vi "Post_Process_Measurement.vi"(1 "Raw data file":path) -> ()   [LabVIEW 2011]
uses:
  Controls/Setup.ctl
  Controls/Post_Process.ctl
  Controls/Save_Data.ctl
  Globals/Constants_global.vi
  Globals/Dynamic_call_global.ph.vi
panel:
  in  "User Specific":refnum<vi>
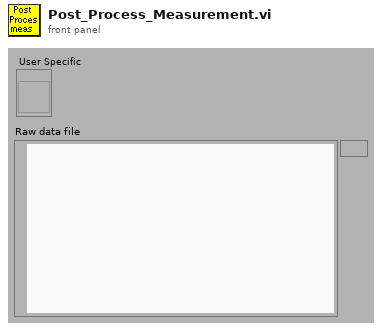
[diagram p1: front panel]
types:
  T1 = enum32{"Bad", "Idle", "Run top level", "Running"}
  T2 = typedef "Setup.ctl" = enum16{"Run Program", "Show Setup", "Save Current Setup", "Setup Front Panel"}
  T3 = typedef "Post_Process.ctl" = enum16{"Take New Data", "Post Process Raw Data File"}
  T4 = typedef "Save_Data.ctl" = enum16{"Save No Data", "Save Data"}
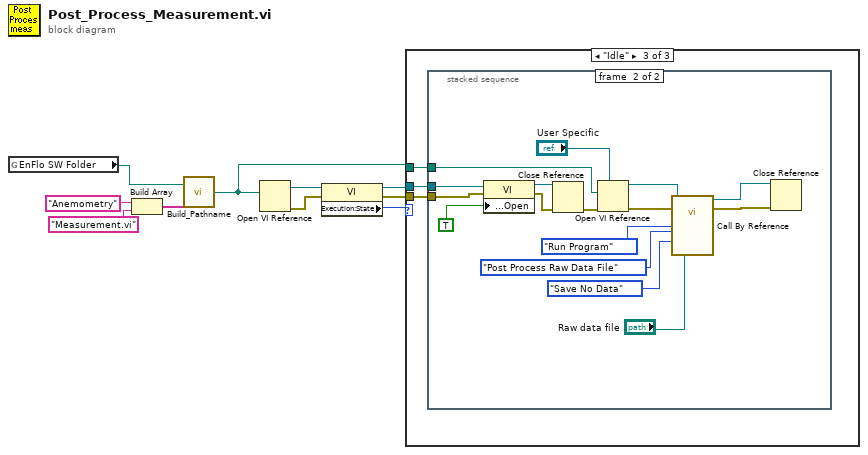
[diagram p0: block diagram]
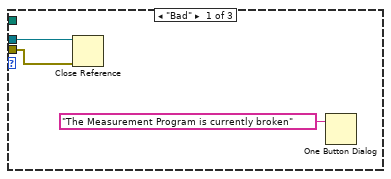
[diagram p2: hidden frame]
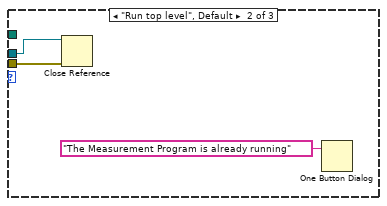
[diagram p3: hidden frame]
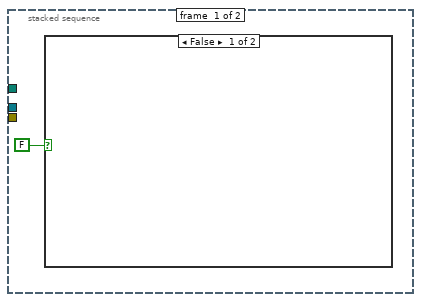
[diagram p4: hidden frame]
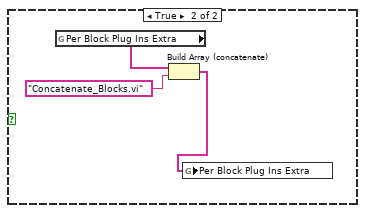
[diagram p5: hidden frame]
diagram:
  n1 = global read "Constants_global.vi" "EnFlo SW Folder"() -> (w10:path)
  n2 = Build Array("Anemometry", "Measurement.vi") -> (w9:string[])
  n3 = call "Build_Pathname.vi"("PathElements"=w9, "PathnameIn"=w10) -> ("AppendedPath"=w1:path)
  n4 = Open VI Reference(vi path=w1) -> (vi reference=w5:refnum<vi>, error out=w6:errorcluster)  [unwired: 1 in, 4 out]
  n5 = property class="VI"(reference=w5, error in=w6) -> (reference out=w3:refnum<vi>, error out=w2:errorcluster, "Execution:State"=w4:T1)
  n6 = case shown="\"Idle\"" w4 {
    tunnel: w3 -> [w12 w15 w19]
    tunnel: w2 -> [w11 w14 w18]
    tunnel: w1 -> [_ _ w17]
    frame "Bad" {
      n7 = Close Reference(reference=w12, error in (no error)=w11) -> ()  [unwired: 1 out]
      n8 = One Button Dialog(message="The Measurement Program is currently broken") -> ()  [unwired: 2 out]
    }
    frame "Run top level", Default {
      n9 = Close Reference(reference=w15, error in (no error)=w14) -> ()  [unwired: 1 out]
      n10 = One Button Dialog(message="The Measurement Program is already running") -> ()  [unwired: 2 out]
    }
    frame "Idle" {
      n11 = stacked-sequence {
        tunnel: w19 -> [_ w39]
        tunnel: w18 -> [_ w38]
        tunnel: w17 -> [_ w27]
        frame #0 {
          n12 = case shown="False" FALSE {
            frame False {
            }
            frame True {
              n13 = global read "Dynamic_call_global.ph.vi" "Per Block Plug Ins Extra"() -> (w23:string[])
              n14 = Build Array (concatenate)(w23, "Concatenate_Blocks.vi") -> (w22:string[])
              n15 = global write "Dynamic_call_global.ph.vi" "Per Block Plug Ins Extra"(w22) -> ()
            }
          }
        }
        frame #1 {
          n16 = property class="VI"(reference=w39, error in=w38, "Front Panel Window:Open"=TRUE) -> (reference out=w30:refnum<vi>, error out=w29:errorcluster)
          n17 = Close Reference(reference=w30, error in (no error)=w29) -> (error out=w28:errorcluster)
          n18 = Open VI Reference(type specifier VI Refnum (for type only)="User Specific", vi path=w27, error in (no error)=w28) -> (vi reference=w25:refnum<vi>, error out=w24:errorcluster)  [unwired: 3 out]
          n19 = call-by-ref "?"(reference=w25, error in=w24, "setup"=Setup."Run Program", "Post Process"=Post_Process."Post Process Raw Data File", "File"=Save_Data."Save No Data", "Raw data file"="Raw data file") -> (reference out=w32:refnum<vi>, error out=w31:errorcluster)  [unwired: 14 in, 2 out]
          n20 = Close Reference(reference=w32, error in (no error)=w31) -> ()  [unwired: 1 out]
        }
      }
    }
  }
